vi "ConfigInputAcquire.vi"(1 "MulticolumnListbox in":refnum<vi>, 3 "ItemNames in":string[][](array[string])) -> (0 "ItemNames out":string[][](array[string]))   [LabVIEW 2018, in "Config.lvlib"]
uses:
  Config.lvlib
panel:
  in  "Replace":bool
  in  "Insert":bool
  in  "Append":bool
  # "Acquire"
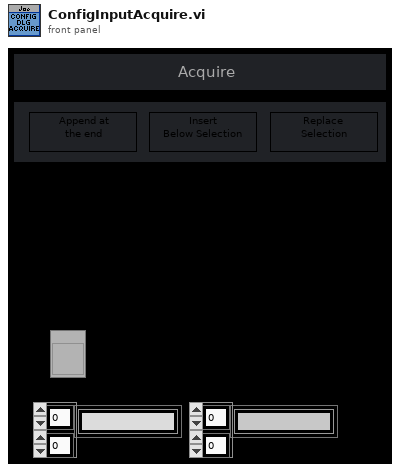
[diagram p1: front panel]
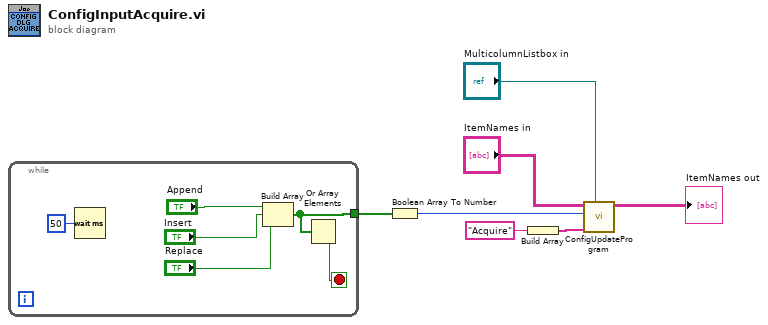
[diagram p0: block diagram]
diagram:
  n1 = while {
    tunnel: [w9] -> w7
    stop <- w10 stop-if-true
    n2 = Wait (ms)(milliseconds to wait=u32 50) -> ()  [unwired: 1 out]
    n3 = Build Array("Append", "Insert", "Replace") -> (w9:bool[])
    n4 = Or Array Elements(Boolean array=w9) -> (logical OR=w10:bool)
  }
  n5 = Boolean Array To Number(Boolean array=w7) -> (number=w6:u32)
  n6 = Build Array("Acquire") -> (w1:string[])
  n7 = call "ConfigUpdateProgram.vi"("MulticolumnListbox in"="MulticolumnListbox in", "New Element"=w1, "Operation"=w6, "ItemNames in"="ItemNames in") -> ("ItemNames out"=→"ItemNames out":string[][])  [unwired: 7 in]
